vi "Initialize TCS.vi"(8 "error in (no error)":errorcluster, 10 "TCS Simulated/Real":bool, 11 "SPARC4_GEI in":refnum<class "SPARC4_GEI.lvclass">) -> (0 "error out":errorcluster, 3 "SPARC4_GEI out":refnum<class "SPARC4_GEI.lvclass">)   [LabVIEW 2018, in "SPARC4_GEI.lvclass"]
uses:
  SPARC4_GEI.lvclass
  SPARC4_GEI.lvclass/SPARC4_GEI.ctl
  TCS/TCS.lvclass
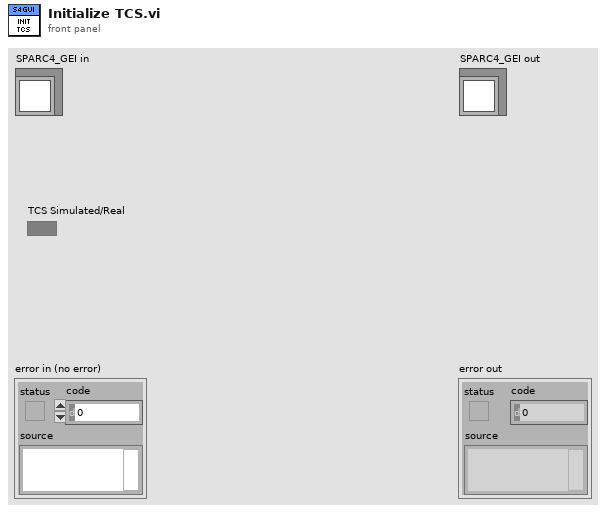
[diagram p1: front panel]
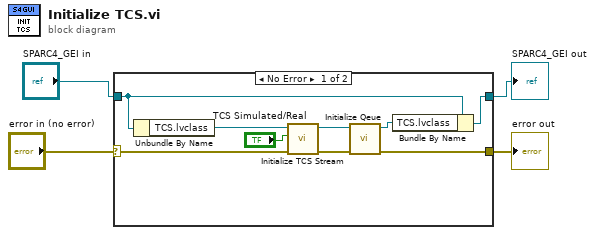
[diagram p0: block diagram]
diagram:
  n1 = case shown="No Error" "error in (no error)" {
    selector: "error in (no error)" -> [w9 w15]
    tunnel: [w6 w15] -> w3
    tunnel: [w13 w14] -> w1
    tunnel: "SPARC4_GEI in" -> [w12 w14]
    frame No Error {
      n2 = Unbundle By Name(w12) -> ("TCS.lvclass"=w8:refnum<class "TCS.lvclass">)
      n3 = call "Initialize TCS Stream.vi"("error in (no error)"=w9, "TCS Simulated/Real"="TCS Simulated/Real", "TCS in"=w8) -> ("error out"=w11:errorcluster, "TCS out"=w10:refnum<class "TCS.lvclass">)  [unwired: 7 in]
      n4 = call "Initialize Qeue.vi"("error in (no error)"=w11, "TCS in"=w10) -> ("error out"=w6:errorcluster, "TCS out"=w7:refnum<class "TCS.lvclass">)  [unwired: 8 in]
      n5 = Bundle By Name(cluster=w12, "TCS.lvclass"=w7) -> (w13:refnum<class "SPARC4_GEI.lvclass">)
    }
    frame Error {
    }
  }
  "error out" <- w3
  "SPARC4_GEI out" <- w1
